vi "Target Vector Shift and Chop.vi"(8 "Learning Gains":T1, 11 "Input Vector":dbl[](array[numeric])) -> (3 "Output Vector":dbl[](array[numeric]))   [LabVIEW 2018, in "COBRA Iterative Learning Control Library.lvlib"]
uses:
  COBRA Iterative Learning Control Library.lvlib
  Target Learning Gains.ctl
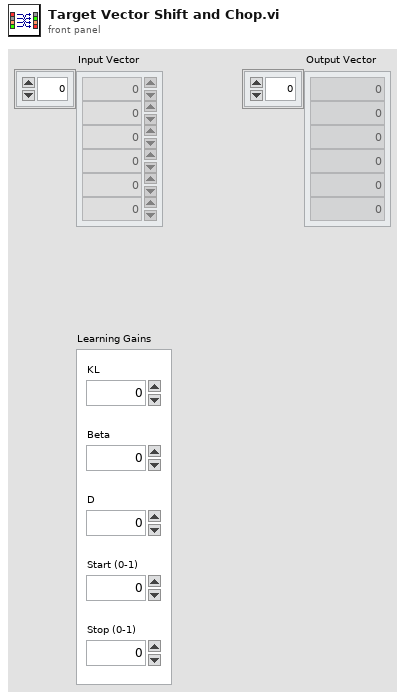
[diagram p1: front panel]
types:
  T1 = typedef "COBRA Iterative Learning Control Library.lvlib/Target Learning Gains.ctl" = cluster{"KL":dbl, "Beta":dbl, "D":i32, "Start (0-1)":dbl, "Stop (0-1)":dbl}
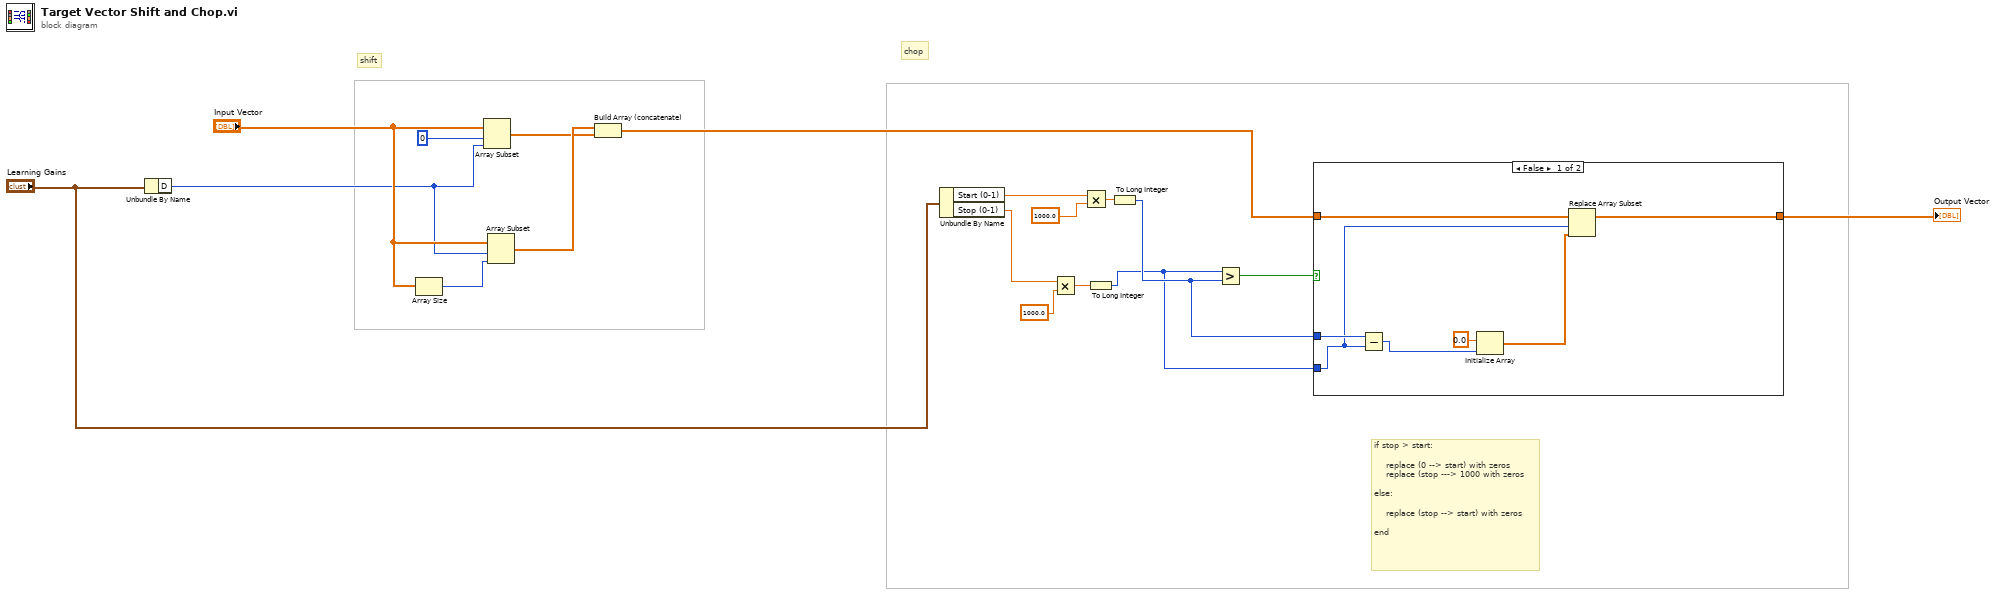
[diagram p0: block diagram]
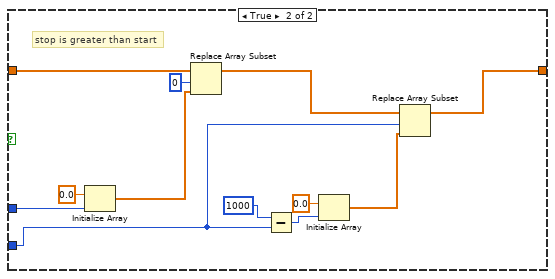
[diagram p2: hidden frame]
diagram:
  # "chop"
  # "if stop > start:\n\n    replace (0 --> start) with zeros\n    replace (stop ---> 1000 with zeros\n\nelse:\n\n    replace (stop --> start) with zeros\n\nend"
  # "shift"
  n1 = Unbundle By Name("Learning Gains") -> ("D"=w13:i32)
  n2 = Array Size(array="Input Vector") -> (size(s)=w16:i32)
  n3 = Array Subset "Array Subset"(array="Input Vector", index=0, length=w13) -> (w14:dbl[])
  n4 = Array Subset "Array Subset"(array="Input Vector", index=w13, length=w16) -> (w15:dbl[])
  n5 = Build Array (concatenate) "Build Array"(w15, w14) -> (w2:dbl[])
  n6 = Unbundle By Name("Learning Gains") -> ("Start (0-1)"=w11:dbl, "Stop (0-1)"=w10:dbl)
  n7 = Multiply(x=w10, y=1000.0) -> (x*y=w6:dbl)
  n8 = Multiply(x=w11, y=1000.0) -> (x*y=w7:dbl)
  n9 = To Long Integer(number=w6) -> (32bit integer=w4:i32)
  n10 = To Long Integer(number=w7) -> (32bit integer=w5:i32)
  n11 = Greater?(x=w4, y=w5) -> (0:w3:bool)
  n12 = case shown="False" w3 {
    tunnel: w2 -> [w22 w37]
    tunnel: w5 -> [w25 w35]
    tunnel: w4 -> [w21 w27]
    tunnel: [w19 w26] -> w1
    frame False {
      n13 = Subtract(x=w25, y=w21) -> (x-y=w24:i32)
      n14 = Initialize Array "Initialize Array"(0.0 ("element"), w24) -> (w20:dbl[])
      n15 = Replace Array Subset "Replace Array Subset"(array=w22, new element=w20, index=w21) -> (w19:dbl[])
    }
    frame True {
      # "stop is greater than start"
      n16 = Initialize Array "Initialize Array"(0.0 ("element"), w35) -> (w34:dbl[])
      n17 = Replace Array Subset "Replace Array Subset"(array=w37, new element=w34, index=0) -> (w29:dbl[])
      n18 = Subtract(x=1000, y=w27) -> (x-y=w31:i32)
      n19 = Initialize Array "Initialize Array"(0.0 ("element"), w31) -> (w28:dbl[])
      n20 = Replace Array Subset "Replace Array Subset"(array=w29, new element=w28, index=w27) -> (w26:dbl[])
    }
  }
  "Output Vector" <- w1
